vi "ConnectToThorlab.vi"(8 "Error In":errorcluster, 11 "Serial Number":string) -> (0 "Error Out":errorcluster, 3 "KCubeDCServo":refnum<k24>)   [LabVIEW 2018, in "Thorlabs.lvlib" / "Thorlabs.lvclass"]
doc: "This vi calls into the .NET DLL's for the Thorlab Kinesis. This connects the specified Serial Number so that the device can be controlled.\n\nIf the serial number specified is not present in the system, then an error will be shown. \n\nThis VI can take upwards of 5 seconds if the initialization routine goes until Timeout.\n\nCreator: Slade Jeppesen\nCreated Date: 09/29/20"
uses:
  Thorlabs.lvclass
  C:/AME Test Engineering/LabVIEW/PPLs/Axis/DLLs/ThorLabs.MotionControl.KCube.DCServoCLI.dll
  PPLs/Axis/DLLs/ThorLabs.MotionControl.KCube.DCServoCLI.dll
  e738033f-0db7-47ca-84e0-b5696862fc1b.vi
  6e68722b-00b0-4e4a-b5a6-ef2ed6c5375a.vi
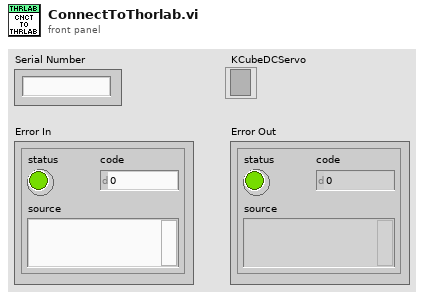
[diagram p1: front panel]
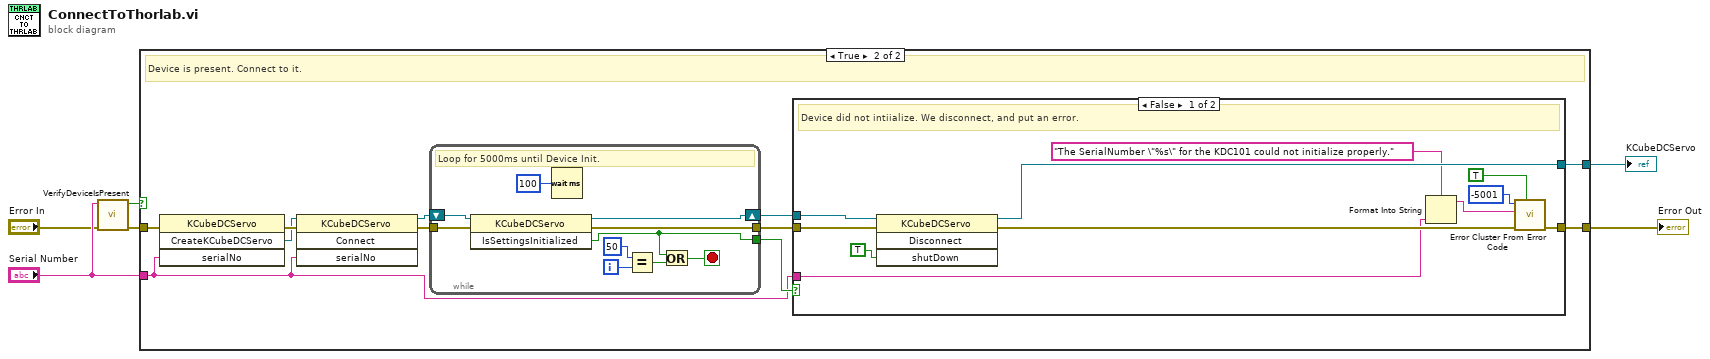
[diagram p0: block diagram]
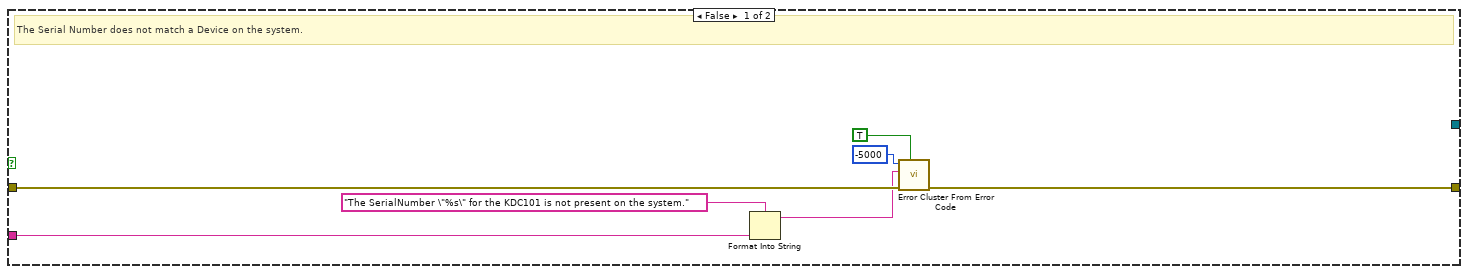
[diagram p2: hidden frame]
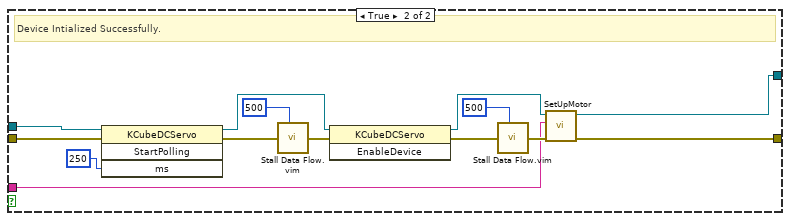
[diagram p3: hidden frame]
diagram:
  n1 = call "VerifyDeviceIsPresent.vi"("Error In"="Error In", "Serial Number in"="Serial Number") -> ("Error Out"=w6:errorcluster, "Present?"=w4:bool)  [unwired: 8 in]
  n2 = case shown="True" w4 {
    tunnel: w6 -> [w13 w17]
    tunnel: [w12 w20] -> w1
    tunnel: [_ w18] -> w5
    tunnel: "Serial Number" -> [w9 w14]
    frame False {
      # "The Serial Number does not match a Device on the system."
      n3 = Format Into String(format string="The SerialNumber \"%s\" for the KDC101 is not present on the system." ("error message (\"\")"), w9) -> (resulting string=w8:string)  [unwired: 2 in, 1 out]
      n4 = call <vilib>:"Error Cluster From Error Code.vi"("show call chain? (False)"=TRUE, "error in (no error)"=w13, "error message (\"\")"=w8, "error code (0)"=-5000) -> ("error out"=w12:errorcluster)  [unwired: 5 in]
    }
    frame True {
      # "Device is present. Connect to it."
      n5 = invoke class="KCubeDCServo" method="CreateKCubeDCServo"(error in=w17, "serialNo"=w14) -> (error out=w16:errorcluster, "CreateKCubeDCServo"=w15:refnum<k24>)  [unwired: 2 in, 2 out]
      n6 = invoke class="KCubeDCServo" method="Connect"(reference=w15, error in=w16, "serialNo"=w14) -> (reference out=w23:refnum<k24>, error out=w24:errorcluster)  [unwired: 1 in, 2 out]
      n7 = while {
        tunnel: w24 -> [w59]
        tunnel: [w53] -> w21
        shift-right: [w52] -> w19
        shift-left: w23 -> [w58]
        tunnel: [w50] -> w22
        i -> [w56]
        stop <- w54 stop-if-true
        # "Loop for 5000ms until Device Init."
        n8 = invoke class="KCubeDCServo" method="IsSettingsInitialized"(reference=w58, error in=w59) -> (reference out=w52:refnum<k24>, error out=w53:errorcluster, "IsSettingsInitialized"=w50:bool)  [unwired: 1 in]
        n9 = Wait (ms)(milliseconds to wait=u32 100) -> ()  [unwired: 1 out]
        n10 = Equal?(x=50, y=w56) -> (x = y?=w51:bool)
        n11 = Or(x=w50, y=w51) -> (x .or. y?=w54:bool)
      }
      n12 = case shown="False" w22 {
        tunnel: w21 -> [w34 w48]
        tunnel: [w28 w37] -> w20
        tunnel: w19 -> [w35 w49]
        tunnel: [w33 w38] -> w18
        tunnel: w14 -> [w27 w39]
        frame False {
          # "Device did not intiialize. We disconnect, and put an error."
          n13 = invoke class="KCubeDCServo" method="Disconnect"(reference=w35, error in=w34, "shutDown"=TRUE) -> (reference out=w33:refnum<k24>, error out=w29:errorcluster)  [unwired: 1 in, 2 out]
          n14 = Format Into String(format string="The SerialNumber \"%s\" for the KDC101 could not initialize properly." ("error message (\"\")"), w27) -> (resulting string=w30:string)  [unwired: 2 in, 1 out]
          n15 = call <vilib>:"Error Cluster From Error Code.vi"("show call chain? (False)"=TRUE, "error in (no error)"=w29, "error message (\"\")"=w30, "error code (0)"=-5001) -> ("error out"=w28:errorcluster)  [unwired: 5 in]
        }
        frame True {
          # "Device Intialized Successfully."
          n16 = invoke class="KCubeDCServo" method="StartPolling"(reference=w49, error in=w48, "ms"=250) -> (reference out=w43:refnum<k24>, error out=w46:errorcluster)  [unwired: 1 in, 2 out]
          n17 = call "Stall Data Flow.vim"("value in"=w46, "milliseconds to wait"=u32 500) -> ("value out"=w44:errorcluster)  [unwired: 1 out]
          n18 = invoke class="KCubeDCServo" method="EnableDevice"(reference=w43, error in=w44) -> (reference out=w36:refnum<k24>, error out=w41:errorcluster)  [unwired: 1 in, 1 out]
          n19 = call "Stall Data Flow.vim"("value in"=w41, "milliseconds to wait"=u32 500) -> ("value out"=w40:errorcluster)  [unwired: 1 out]
          n20 = call "SetUpMotor.vi"("Error In"=w40, "Serial Number"=w39, "KCubeDCServo in"=w36) -> ("Error Out"=w37:errorcluster, "KCubeDCServo out"=w38:refnum<k24>)  [unwired: 7 in]
        }
      }
    }
  }
  "KCubeDCServo" <- w5
  "Error Out" <- w1
